vi "Main.vi"() -> ()   [LabVIEW 2016]
uses:
  Experiment States.ctl
  <vilib>/DAQmx/read.llb/DAQmx Read (Analog 2D DBL NChan NSamp).vi
  <vilib>/DAQmx/miscellaneous.llb/DAQmx Fill In Error Info.vi
  <vilib>/DAQmx/write.llb/DAQmx Write (Analog DBL 1Chan 1Samp).vi
panel:
  in  "Cooling Water Control Channel":tag
  in  "Condensate Flow Rate 2 Channel":tag
  in  "Condensate Flow Rate 1 Channel":tag
  in  "Cooling Water Flow Rate Channel":tag
  in  "Steam Pressure Channel":tag="cDAQ2Mod4/ai0"
  out "Condensate Flow Rate 2":dbl(knob) scale=0.0..10.0
  out "Condensate Flow Rate Graph 2":cluster{"X":dbl, "Y":dbl}[](graph)
  out "Condensate Flow Rate Graph 1":cluster{"X":dbl, "Y":dbl}[](graph)
  out "Condensate Flow Rate 1":dbl(knob) scale=0.0..10.0
  in  "Cooling Water Control Valve (% Closed)":dbl(slide) scale=0.0..100.0
  out "Cooling Water Flow Rate (gpm)":dbl(knob) scale=0.0..10.0
  out "Steam Pressure (psig)":dbl(knob)=-0.002836266400000001 scale=0.0..5.0
  out "Current Time (seconds)":dbl=43.003
  out "Lower Condensate Tube":dbl(slide)=22.801415634118047 scale=0.0..100.0
  out "Upper Condensate Tube":dbl(slide)=22.55227574910883 scale=0.0..100.0
  out "Inlet Steam":dbl(slide)=22.777040196136387 scale=0.0..100.0
  out "Condenser Tube Glass":dbl(slide)=22.73286738210012 scale=0.0..100.0
  out "Total Condensate":dbl(slide)=22.772184277137242 scale=0.0..100.0
  out "Exhaust Cooling Water":dbl(slide)=22.347402721961156 scale=0.0..100.0
  out "Inlet Cooling Water":dbl(slide)=22.935723539384863 scale=0.0..100.0
  out "Exhaust Cooling Water Graph":cluster{"X":dbl, "Y":dbl}[](graph)
  in  "Thermocouple 13 Channel":tag="cDAQ2Mod1/ai13"
  in  "Thermocouple 12 Channel":tag="cDAQ2Mod1/ai12"
  in  "Thermocouple 11 Channel":tag="cDAQ2Mod1/ai11"
  in  "Thermocouple 10 Channel":tag="cDAQ2Mod1/ai10"
  in  "Thermocouple 9 Channel":tag="cDAQ2Mod1/ai9"
  in  "Thermocouple 8 Channel":tag="cDAQ2Mod1/ai8"
  in  "Thermocouple 7 Channel":tag="cDAQ2Mod1/ai7"
  in  "End Experiment?":bool
  in  "Start":bool
  # "Thermocouple Key:\n7) Inlet Cooling Water\n8) Exhaust Cooling Water\n9) Total Condensate\n10) Condenser Tube Glass\n11) Inlet Steam\n12) Upper Condensate Tube\n13) Lower Condensate Tube"
  # "HORIZONTAL STEAM CONDENSATION"
  # "Choose  Channels before starting the experiment!"
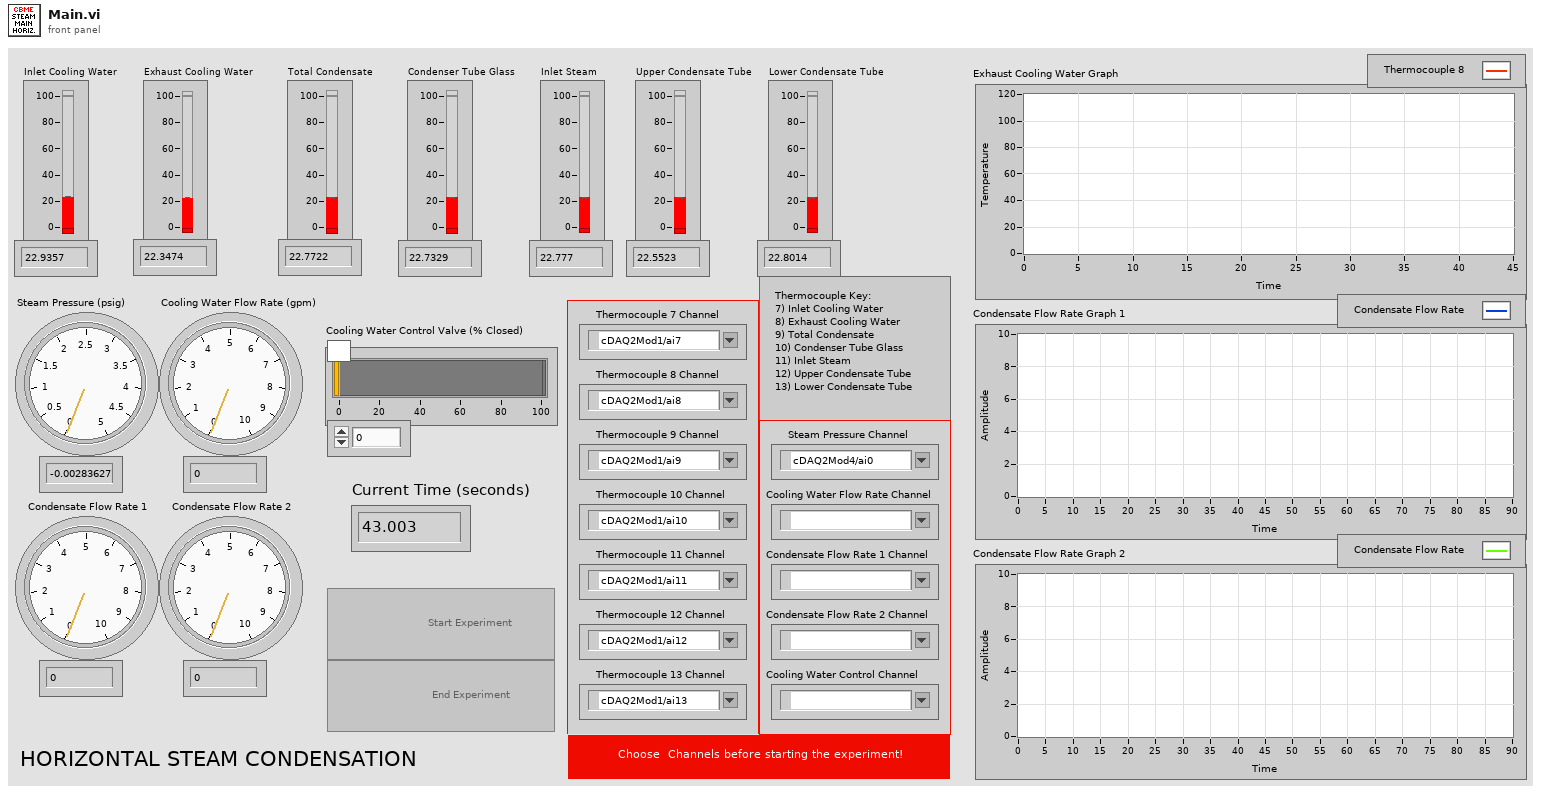
[diagram p1: front panel]
types:
  T1 = typedef "Experiment States.ctl" = enum16{"Setup", "Data Collection", "Export", "Finish"}
  T2 = enum8{"Enabled", "Disabled", "Disabled and Grayed Out"}
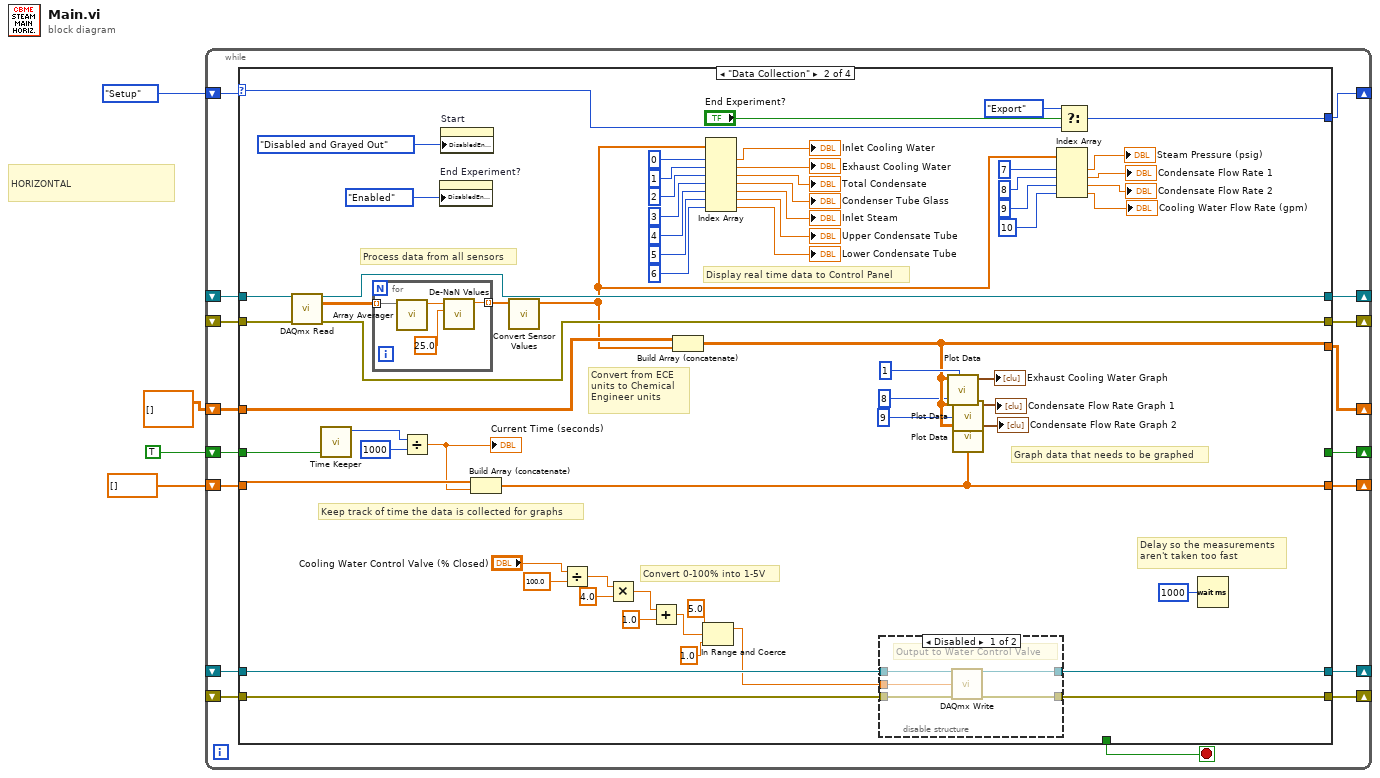
[diagram p0: block diagram]
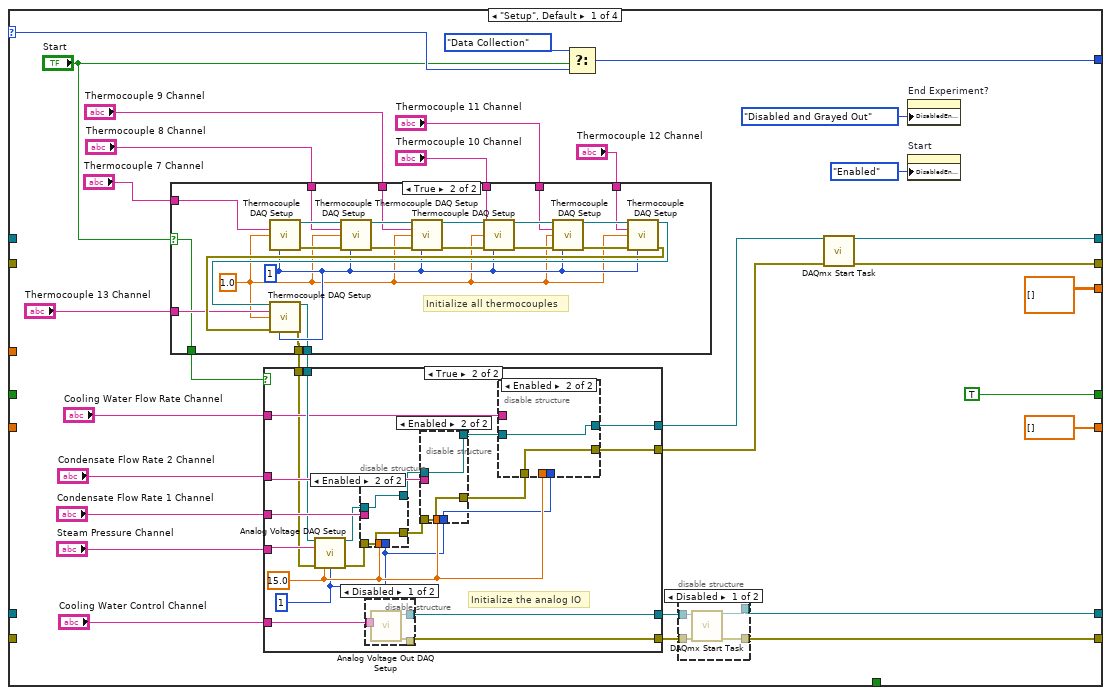
[diagram p2: hidden frame]
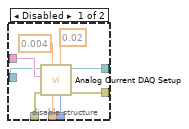
[diagram p6: hidden frame]
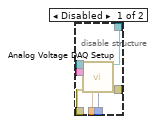
[diagram p7: hidden frame]
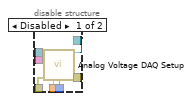
[diagram p8: hidden frame]
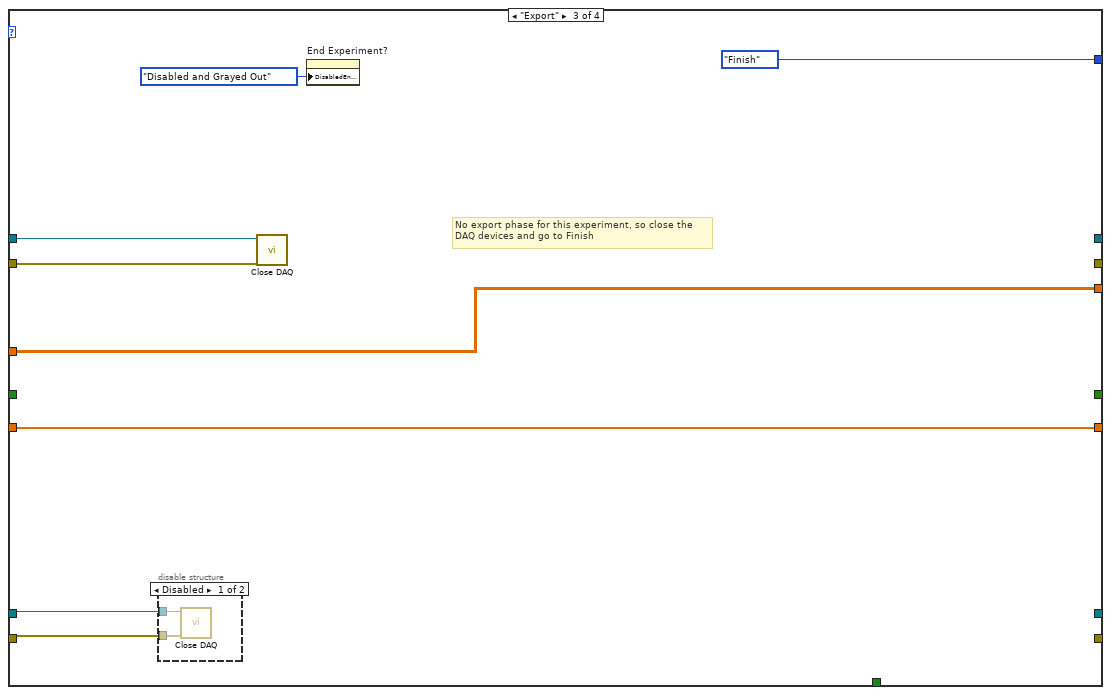
[diagram p11: hidden frame]
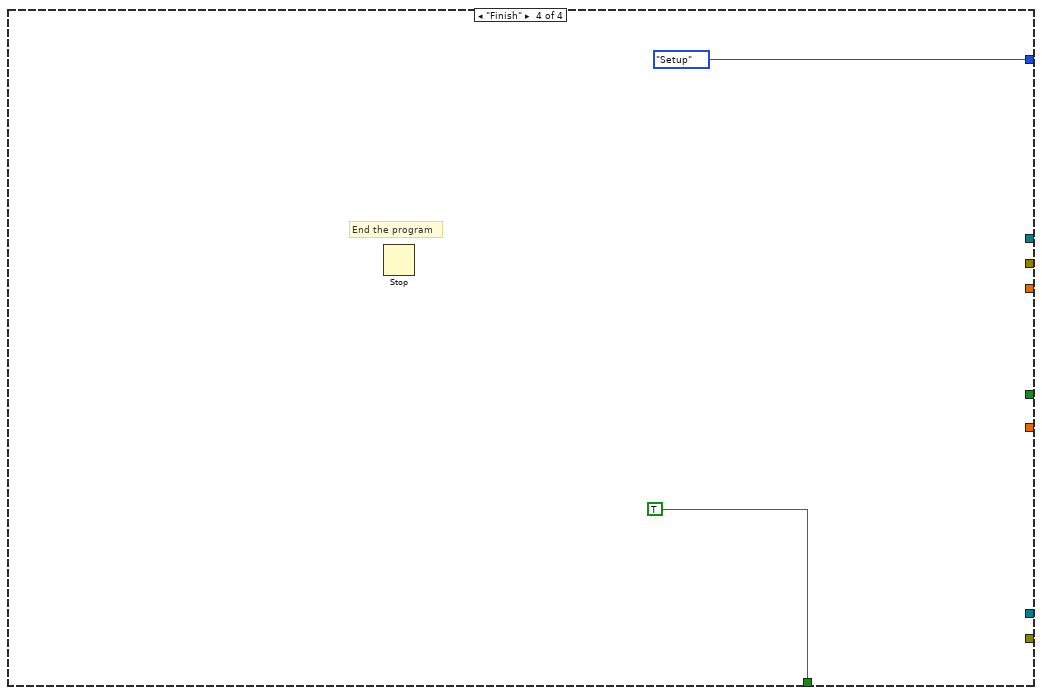
[diagram p13: hidden frame]
diagram:
  # "HORIZONTAL"
  n1 = while {
    shift-right: [w9] -> _
    shift-left: Experiment_States."Setup" ("Enum") -> [w21]
    shift-right: [w18] -> _
    shift-left: _ -> [w16]
    shift-right: [w19] -> _
    shift-left: _ -> [w17]
    shift-right: [w15] -> _
    shift-left: dbl[][] [] -> [w14]
    shift-right: [w10] -> _
    shift-left: TRUE ("Reset?") -> [w13]
    shift-right: [w11] -> _
    shift-left: dbl[] [] -> [w12]
    shift-right: [w8] -> _
    shift-left: _ -> [w6]
    shift-right: [w7] -> _
    shift-left: _ -> [w5]
    stop <- w20 stop-if-true
    n2 = case shown="\"Data Collection\"" w21 {
      selector: w21 -> [w53 w195 _ _]
      tunnel: [w51 w197 Experiment_States."Finish" ("Enum") Experiment_States."Setup" ("Enum")] -> w9
      tunnel: [_ _ _ TRUE] -> w20
      tunnel: [w43 w169 _ _] -> w19
      tunnel: [w42 w168 _ _] -> w18
      tunnel: w17 -> [_ w193 w211 _]
      tunnel: w16 -> [_ w192 w210 _]
      tunnel: [dbl[][] [] w159 w212 _] -> w15
      tunnel: w14 -> [_ w177 w212 _]
      tunnel: w13 -> [_ w176 _ _]
      tunnel: w12 -> [_ w172 w213 _]
      tunnel: [dbl[] [] w160 w213 _] -> w11
      tunnel: [TRUE ("Reset?") _ _ _] -> w10
      tunnel: [w24 w150 _ _] -> w8
      tunnel: [w23 w149 _ _] -> w7
      tunnel: w6 -> [_ w152 w208 _]
      tunnel: w5 -> [_ w151 w207 _]
      frame "Setup", Default {
        n3 = case shown="True" "Start" {
          selector: "Start" -> [w109 w111]
          tunnel: "Thermocouple 7 Channel" -> [_ w121]
          tunnel: "Thermocouple 8 Channel" -> [_ w120]
          tunnel: "Thermocouple 9 Channel" -> [_ w119]
          tunnel: "Thermocouple 10 Channel" -> [_ w118]
          tunnel: "Thermocouple 11 Channel" -> [_ w117]
          tunnel: "Thermocouple 12 Channel" -> [_ w116]
          tunnel: "Thermocouple 13 Channel" -> [_ w115]
          tunnel: [_ w112] -> w31
          tunnel: [w109 w111] -> w27
          tunnel: [_ w110] -> w22
          frame False {
          }
          frame True {
            w113 = 1.0 ("Sample Rate")
            w114 = 1 ("samples per channel")
            # "Initialize all thermocouples"
            n4 = call "Thermocouple DAQ Setup.vi"("physical channels"=w121, "Sample Rate"=w113, "samples per channel"=w114) -> ("task out"=w122:refnum<k21>, "error out"=w133:errorcluster)  [unwired: 11 in]
            n5 = call "Thermocouple DAQ Setup.vi"("task in"=w122, "physical channels"=w120, "Sample Rate"=w113, "error in"=w133, "samples per channel"=w114) -> ("task out"=w123:refnum<k21>, "error out"=w132:errorcluster)  [unwired: 9 in]
            n6 = call "Thermocouple DAQ Setup.vi"("task in"=w123, "physical channels"=w119, "Sample Rate"=w113, "error in"=w132, "samples per channel"=w114) -> ("task out"=w124:refnum<k21>, "error out"=w131:errorcluster)  [unwired: 9 in]
            n7 = call "Thermocouple DAQ Setup.vi"("task in"=w124, "physical channels"=w118, "Sample Rate"=w113, "error in"=w131, "samples per channel"=w114) -> ("task out"=w125:refnum<k21>, "error out"=w130:errorcluster)  [unwired: 9 in]
            n8 = call "Thermocouple DAQ Setup.vi"("task in"=w125, "physical channels"=w117, "Sample Rate"=w113, "error in"=w130, "samples per channel"=w114) -> ("task out"=w126:refnum<k21>, "error out"=w129:errorcluster)  [unwired: 9 in]
            n9 = call "Thermocouple DAQ Setup.vi"("task in"=w126, "physical channels"=w116, "Sample Rate"=w113, "error in"=w129, "samples per channel"=w114) -> ("task out"=w127:refnum<k21>, "error out"=w128:errorcluster)  [unwired: 9 in]
            n10 = call "Thermocouple DAQ Setup.vi"("task in"=w127, "physical channels"=w115, "Sample Rate"=w113, "error in"=w128, "samples per channel"=w114) -> ("task out"=w112:refnum<k21>, "error out"=w110:errorcluster)  [unwired: 9 in]
          }
        }
        n11 = case shown="True" w27 {
          tunnel: "Cooling Water Control Channel" -> [_ w76]
          tunnel: "Steam Pressure Channel" -> [_ w75]
          tunnel: "Condensate Flow Rate 1 Channel" -> [_ w74]
          tunnel: "Condensate Flow Rate 2 Channel" -> [_ w73]
          tunnel: [_ w72] -> w26
          tunnel: w31 -> [_ w71]
          tunnel: "Cooling Water Flow Rate Channel" -> [_ w70]
          tunnel: [_ w69] -> w29
          tunnel: [_ w68] -> w28
          tunnel: [_ w67] -> w25
          tunnel: w22 -> [_ w66]
          frame False {
          }
          frame True {
            w59 = 1 ("samples per channel")
            w60 = 15.0 ("Sample Rate")
            # "Initialize the analog IO"
            n12 = call "Analog Voltage DAQ Setup.vi"("task in"=w71, "physical channels"=w75, "error in"=w66, "Sample Rate"=w60, "samples per channel"=w59) -> ("task out"=w65:refnum<k21>, "error out"=w63:errorcluster)  [unwired: 9 in]
            n13 = disable-structure shown="Enabled" {
              disable-tunnel: w74 -> [w106 _]
              disable-tunnel: w65 -> [w105 w108]
              disable-tunnel: [w104 w108] -> w64
              disable-tunnel: w63 -> [w103 w107]
              disable-tunnel: [w102 w107] -> w62
              disable-tunnel: w60 -> [w101 _]
              disable-tunnel: w59 -> [w100 _]
              frame Disabled {
                n14 = call "Analog Voltage DAQ Setup.vi"("task in"=w105, "physical channels"=w106, "error in"=w103, "Sample Rate"=w101, "samples per channel"=w100) -> ("task out"=w104:refnum<k21>, "error out"=w102:errorcluster)  [unwired: 9 in]
              }
              frame Enabled {
              }
            }
            n15 = disable-structure shown="Disabled" {
              disable-tunnel: w76 -> [w79 _]
              disable-tunnel: [w78 _] -> w72
              disable-tunnel: [w77 _] -> w67
              frame Disabled {
                n16 = call "Analog Voltage Out DAQ Setup.vi"("physical channels"=w79) -> ("error out"=w77:errorcluster, "task out"=w78:refnum<k21>)  [unwired: 9 in]
              }
              frame Enabled {
              }
            }
            n17 = disable-structure shown="Enabled" {
              disable-tunnel: w73 -> [w97 _]
              disable-tunnel: w64 -> [w96 w99]
              disable-tunnel: w62 -> [w95 w98]
              disable-tunnel: [w94 w99] -> w61
              disable-tunnel: w60 -> [w93 _]
              disable-tunnel: w59 -> [w92 _]
              disable-tunnel: [w91 w98] -> w58
              frame Disabled {
                n18 = call "Analog Voltage DAQ Setup.vi"("task in"=w96, "physical channels"=w97, "error in"=w95, "Sample Rate"=w93, "samples per channel"=w92) -> ("task out"=w94:refnum<k21>, "error out"=w91:errorcluster)  [unwired: 9 in]
              }
              frame Enabled {
              }
            }
            n19 = disable-structure shown="Enabled" {
              disable-tunnel: w70 -> [w88 _]
              disable-tunnel: [w87 w89] -> w69
              disable-tunnel: [w86 w90] -> w68
              disable-tunnel: w61 -> [w85 w90]
              disable-tunnel: w60 -> [w82 _]
              disable-tunnel: w59 -> [w81 _]
              disable-tunnel: w58 -> [w80 w89]
              frame Disabled {
                n20 = call "Analog Current DAQ Setup.vi"("samples per channel"=w81, "minimum value"=0.02, "rate"=w82, "maximum value"=0.004, "error in"=w80, "physical channels"=w88, "task in"=w85) -> ("error out"=w87:errorcluster, "task out"=w86:refnum<k21>)  [unwired: 3 in]
              }
              frame Enabled {
              }
            }
          }
        }
        n21 = Select(t=Experiment_States."Data Collection", s="Start", f=w53) -> (s? t:f=w51:T1)
        n22 = disable-structure shown="Disabled" {
          disable-tunnel: w26 -> [w57 _]
          disable-tunnel: w25 -> [w56 _]
          disable-tunnel: [w55 _] -> w24
          disable-tunnel: [w54 _] -> w23
          frame Disabled {
            n23 = call <vilib>:"DAQmx Start Task.vi"("task/channels in"=w57, "error in"=w56) -> ("task out"=w55:refnum<k21>, "error out"=w54:errorcluster)  [unwired: 12 in]
          }
          frame Enabled {
          }
        }
        n24 = call <vilib>:"DAQmx Start Task.vi"("task/channels in"=w28, "error in"=w29) -> ("task out"=w43:refnum<k21>, "error out"=w42:errorcluster)  [unwired: 12 in]
        n25 = property on="End Experiment?" class="Bool"("DisabledEnum"=T2."Disabled and Grayed Out" ("Disabled")) -> ()  [unwired: 2 in, 2 out]
        n26 = property on="Start" class="Bool"("DisabledEnum"=T2."Enabled" ("Disabled")) -> ()  [unwired: 2 in, 2 out]
      }
      frame "Data Collection" {
        # "Convert from ECE \nunits to Chemical \nEngineer units"
        # "Delay so the measurements\naren't taken too fast"
        # "Keep track of time the data is collected for graphs"
        # "Graph data that needs to be graphed"
        # "Display real time data to Control Panel"
        # "Process data from all sensors"
        # "Convert 0-100% into 1-5V"
        n27 = call-poly <vilib>:"DAQmx Read.vi"("task/channels in"=w193, "error in"=w192) -> ("task out"=w169:refnum<k21>, "data"=w191:dbl[][], "error out"=w168:errorcluster)  [unwired: 11 in]
        n28 = call "Time Keeper.vi"("Reset?"=w176) -> ("Time Elapsed (ms)"=w175:u32)  [unwired: 10 in]
        n29 = for {
          tunnel: w191 -> [w203] mode=indexing
          tunnel: [w204] -> w164 mode=indexing
          n30 = call "Array Averager.vi"("Array"=w203) -> ("Averaged Array"=w206:dbl)  [unwired: 10 in]
          n31 = call "De-NaN Values.vi"("Last Valid"=25.0, "Input"=w206) -> ("De-NaN"=w204:dbl)  [unwired: 9 in]
        }
        n32 = Divide(x=w175, y=u32 1000) -> (x/y=w167:dbl)
        "Current Time (seconds)" <- w167
        n33 = property on="End Experiment?" class="Bool"("DisabledEnum"=T2."Enabled" ("Disabled")) -> ()  [unwired: 2 in, 2 out]
        n34 = property on="Start" class="Bool"("DisabledEnum"=T2."Disabled and Grayed Out" ("Disabled")) -> ()  [unwired: 2 in, 2 out]
        n35 = Build Array (concatenate)(w172, w167) -> (w160:dbl[])
        n36 = call "Convert Sensor Values.vi"("ECE Units"=w164) -> ("CBME Units"=w134:dbl[])  [unwired: 10 in]
        n37 = Divide(x="Cooling Water Control Valve (% Closed)", y=100.0) -> (x/y=w156:dbl)
        n38 = Multiply(x=w156, y=4.0) -> (x*y=w154:dbl)
        n39 = Add(x=w154, y=1.0) -> (x+y=w147:dbl)
        n40 = Build Array (concatenate)(w177, w134) -> (w159:dbl[][])
        n41 = In Range and Coerce(upper limit=5.0, x=w147, lower limit=1.0) -> (coerced(x)=w148:dbl)  [unwired: 1 out]
        n42 = Index Array(array=w134, index #1=0 ("index"), index #2=1 ("index"), index #3=2 ("index"), index #4=3 ("index"), index #5=4 ("index"), index #6=5 ("index"), index #7=6 ("index")) -> (element #1=→"Inlet Cooling Water":dbl, element #2=→"Exhaust Cooling Water":dbl, element #3=→"Total Condensate":dbl, element #4=→"Condenser Tube Glass":dbl, element #5=→"Inlet Steam":dbl, element #6=→"Upper Condensate Tube":dbl, element #7=→"Lower Condensate Tube":dbl)
        n43 = disable-structure shown="Disabled" {
          disable-tunnel: w152 -> [w202 _]
          disable-tunnel: w151 -> [w201 _]
          disable-tunnel: [w200 _] -> w150
          disable-tunnel: [w199 _] -> w149
          disable-tunnel: w148 -> [w198 _]
          frame Disabled {
            # "Output to Water Control Valve"
            n44 = call-poly <vilib>:"DAQmx Write.vi"("task/channels in"=w202, "data"=w198, "error in"=w201) -> ("task out"=w200:refnum<k21>, "error out"=w199:errorcluster)  [unwired: 10 in, 1 out]
          }
          frame Enabled {
          }
        }
        n45 = call "Plot Data.vi"("Time Array"=w160, "Device ID (0 index)"=1 ("thermocouple (0 index)"), "Data Array"=w159) -> ("Graph"=→"Exhaust Cooling Water Graph":cluster{"X":dbl, "Y":dbl}[])  [unwired: 8 in]
        n46 = call "Plot Data.vi"("Time Array"=w160, "Device ID (0 index)"=8, "Data Array"=w159) -> ("Graph"=→"Condensate Flow Rate Graph 1":cluster{"X":dbl, "Y":dbl}[])  [unwired: 8 in]
        n47 = call "Plot Data.vi"("Time Array"=w160, "Device ID (0 index)"=9, "Data Array"=w159) -> ("Graph"=→"Condensate Flow Rate Graph 2":cluster{"X":dbl, "Y":dbl}[])  [unwired: 8 in]
        n48 = Index Array(array=w134, index #1=7 ("index"), index #2=8 ("index"), index #3=9 ("index"), index #4=10 ("index")) -> (element #1=→"Steam Pressure (psig)":dbl, element #2=→"Condensate Flow Rate 1":dbl, element #3=→"Condensate Flow Rate 2":dbl, element #4=→"Cooling Water Flow Rate (gpm)":dbl)
        n49 = Select(t=Experiment_States."Export", s="End Experiment?", f=w195) -> (s? t:f=w197:T1)
        n50 = Wait (ms)(milliseconds to wait=u32 1000) -> ()  [unwired: 1 out]
      }
      frame "Export" {
        # "No export phase for this experiment, so close the\nDAQ devices and go to Finish"
        n51 = disable-structure shown="Disabled" {
          disable-tunnel: w208 -> [w216 _]
          disable-tunnel: w207 -> [w215 _]
          frame Disabled {
            n52 = call "Close DAQ.vi"("error in (no error)"=w215, "Refnum in"=w216) -> ()  [unwired: 10 in]
          }
          frame Enabled {
          }
        }
        n53 = call "Close DAQ.vi"("error in (no error)"=w210, "Refnum in"=w211) -> ()  [unwired: 10 in]
        n54 = property on="End Experiment?" class="Bool"("DisabledEnum"=T2."Disabled and Grayed Out" ("Disabled")) -> ()  [unwired: 2 in, 2 out]
      }
      frame "Finish" {
        # "End the program"
        n55 = Stop() -> ()  [unwired: 1 in]
      }
    }
  }
